vi "Lookup Amount per Color.vi"(10 "All":T1(array[cluster]), 11 "Search":cluster{"Amount":i32, "Color":string}) -> (3 "Numeric":i32)   [LabVIEW 2018]
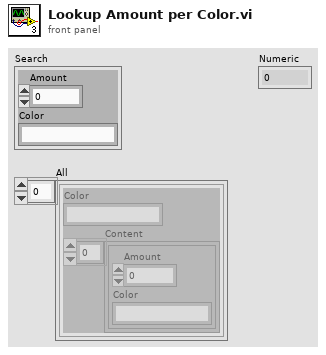
[diagram p1: front panel]
types:
  T1 = cluster{"Color":string, "Content":cluster{"Amount":i32, "Color":string}[]}[]
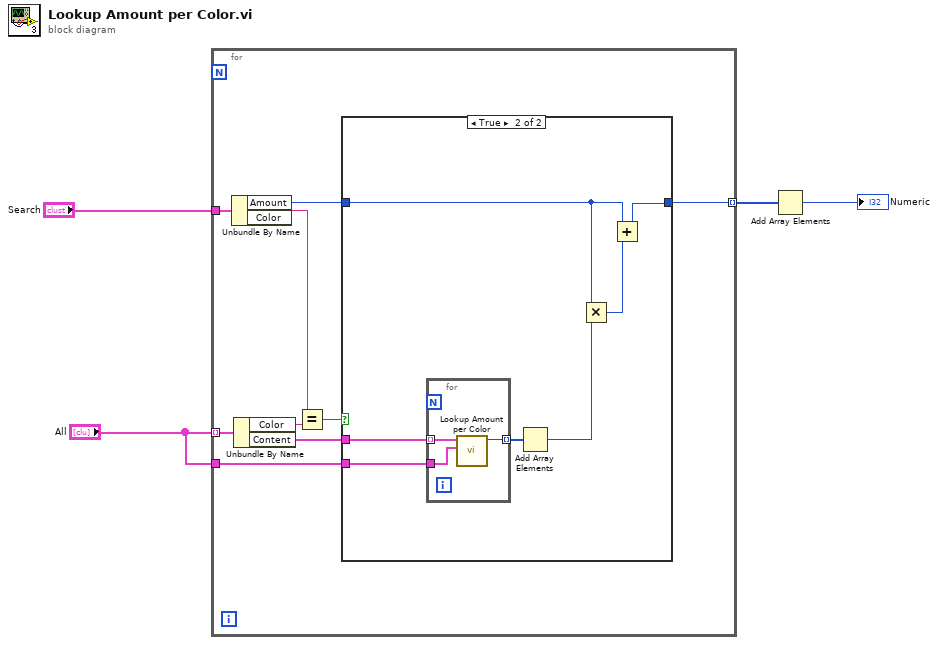
[diagram p0: block diagram]
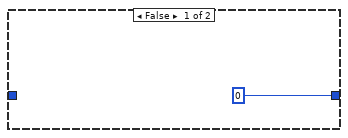
[diagram p2: hidden frame]
diagram:
  n1 = for {
    tunnel: "All" -> [w13] mode=indexing
    tunnel: "Search" -> [w11]
    tunnel: [w6] -> w2 mode=indexing
    tunnel: "All" -> [w5]
    n2 = Unbundle By Name(w11) -> ("Amount"=w7:i32, "Color"=w8:string)
    n3 = Unbundle By Name(w13) -> ("Color"=w12:string, "Content"=w9:cluster{"Amount":i32, "Color":string}[])
    n4 = Equal?(x=w8, y=w12) -> (x = y?=w10:bool)
    n5 = case shown="True" w10 {
      tunnel: w9 -> [_ w19]
      tunnel: w7 -> [_ w18]
      tunnel: [0 w16] -> w6
      tunnel: w5 -> [_ w21]
      frame False {
      }
      frame True {
        n6 = for {
          tunnel: w19 -> [w24] mode=indexing
          tunnel: w21 -> [w23]
          tunnel: [w22] -> w15 mode=indexing
          n7 = call "Lookup Amount per Color.vi"("All"=w23, "Search"=w24) -> ("Numeric"=w22:i32)  [unwired: 9 in]
        }
        n8 = Add Array Elements(numeric array=w15) -> (sum=w20:i32)
        n9 = Multiply(x=w18, y=w20) -> (x*y=w17:i32)
        n10 = Add(x=w18, y=w17) -> (x+y=w16:i32)
      }
    }
  }
  n11 = Add Array Elements(numeric array=w2) -> (sum=→"Numeric":i32)
